vi "dIMU Complimentary Filter.vi"(7 "Port":T2 items=["Port 1", "Port 2", "Port 3", "Port 4"], 9 "Tau":dbl=3.0, 11 "NXT":T1) -> (0 "Yaw (deg)":dbl, 1 "Roll (deg)":dbl, 2 "Pitch (deg)":dbl, 3 "NXT":T1={"Hardware"="NXT", "Flattened String"=""})   [LabVIEW 2010]
uses:
  <vilib>/NXT/Block Support/NXT_InputPort.ctl
  <vilib>/NXT/Subs/LVHSConnector.ctl
  subVIs/dIMU_Accel_gs.vi
  subVIs/dIMU_Gyro_rads.vi
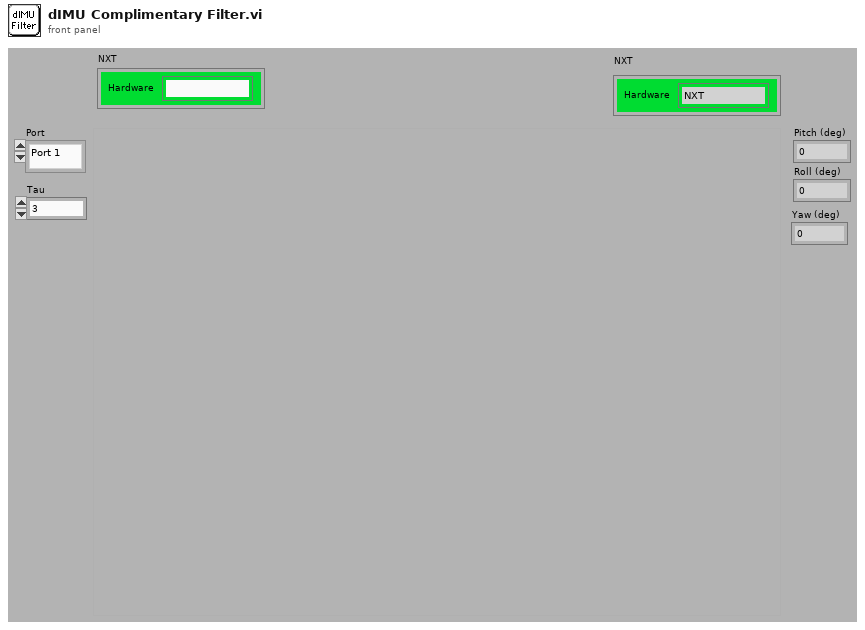
[diagram p1: front panel]
types:
  T1 = typedef "LVHSConnector.ctl" = cluster{"Hardware":string, "Flattened String":string}
  T2 = typedef "NXT_InputPort.ctl" = u8
  T3 = cluster{"Z Accel Offset":dbl, "Y Accel Offset":dbl, "X Accel Offset":dbl, "Z Gyro Offset":dbl, "Y Gyro Offset":dbl, "X Gyro Offset":dbl}
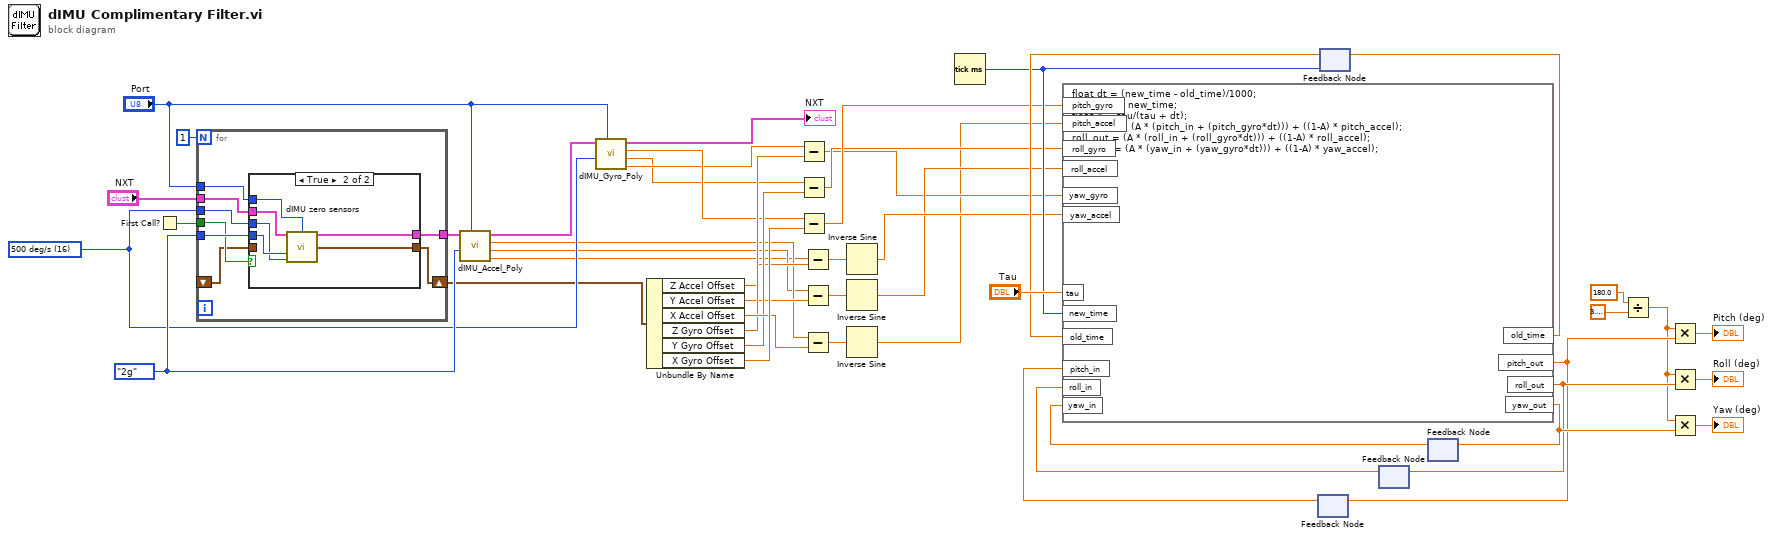
[diagram p0: block diagram]
diagram:
  w18 = u8 16 items=["250 deg/s"=0, "500 deg/s"=16, "2000 deg/s"=32] ("Gyro Scale")
  w24 = enum8{"2g", "4g", "8g"}."2g" ("Maximum Range")
  # "current axes are pitch (x) forward, roll (y) left, and yaw (z) up,\nshould these be rotated to standard aviation axes?"
  # "y = f(x) = A * y + (1-A) * x\nA = tau/(tau + dt)"
  n1 = First Call?() -> (First Call?: T/F=w17:bool)
  n2 = for {
    N: 1 -> [_]
    tunnel: "NXT" -> [w55]
    tunnel: [w54] -> w26
    tunnel: "Port" -> [w53]
    tunnel: w24 -> [w52]
    tunnel: w18 -> [w51]
    tunnel: w17 -> [w50]
    shift-right: [w49] -> w15
    shift-left: _ -> [w48]
    n3 = case shown="True" w50 {
      tunnel: w55 -> [w57 w63]
      tunnel: [w57 w62] -> w54
      tunnel: w53 -> [_ w61]
      tunnel: w52 -> [_ w60]
      tunnel: w51 -> [_ w59]
      tunnel: [w56 w58] -> w49
      tunnel: w48 -> [w56 _]
      frame False {
      }
      frame True {
        n4 = call "dIMU zero sensors.vi"("NXT 2"=w63, "Port"=w61, "Maximum Range"=w60, "Gyro Scale"=w59) -> ("NXT"=w62:T1, "Sensor Offsets"=w58:T3)  [unwired: 10 in]
      }
    }
  }
  n5 = call-poly "dIMU_Accel_Poly.vi"("Port"="Port", "Maximum Range"=w24, "NXT"=w26) -> ("Z Accel (g)"=w4:dbl, "Y Accel (g)"=w5:dbl, "X Accel (g)"=w6:dbl, "NXT"=w47:T1)  [unwired: 5 in]
  n6 = call-poly "dIMU_Gyro_Poly.vi"("Port"="Port", "Gyro Scale"=w18, "NXT"=w47) -> ("Z Gyro (rad/s"=w2:dbl, "Y Gyro (rad/s)"=w1:dbl, "X Gyro (rad/s)"=w3:dbl, "NXT"=→"NXT":T1)  [unwired: 5 in]
  n7 = Unbundle By Name(w15) -> ("Z Accel Offset"=w7:dbl, "Y Accel Offset"=w8:dbl, "X Accel Offset"=w12:dbl, "Z Gyro Offset"=w9:dbl, "Y Gyro Offset"=w10:dbl, "X Gyro Offset"=w14:dbl)
  n8 = Subtract(x=w2, y=w9) -> (x-y=w19:dbl)
  n9 = Subtract(x=w1, y=w10) -> (x-y=w20:dbl)
  n10 = Subtract(x=w3, y=w14) -> (x-y=w21:dbl)
  n11 = Subtract(x=w4, y=w7) -> (x-y=w22:dbl)
  n12 = Subtract(x=w5, y=w8) -> (x-y=w23:dbl)
  n13 = Subtract(x=w6, y=w12) -> (x-y=w11:dbl)
  n14 = Inverse Sine(1:w22) -> (0:w41:dbl)
  n15 = Inverse Sine(1:w23) -> (0:w40:dbl)
  n16 = Inverse Sine(1:w11) -> (0:w13:dbl)
  n17 = Tick Count (ms)() -> (millisecond timer value=w42:u32)
  n18 = feedback #1() -> (w29:dbl)  [unwired: 1 in]
  n19 = feedback #2(w42) -> (w43:dbl)
  n20 = feedback #3() -> (w31:dbl)  [unwired: 1 in]
  n21 = feedback #4() -> (w33:dbl)  [unwired: 1 in]
  n22 = formula code="float dt = (new_time - old_time)/1000;\nold_time = new_time;\nfloat A = tau/(tau + dt);\npitch_out = (A * (pitch_in + (pitch_gyro*dt))) + ((1-A) * pitch_accel);\nroll_out = (A * (roll_in + (roll_gyro*dt))) + ((1-A) * roll_accel);\nyaw_out = (A * (yaw_in + (yaw_gyro*dt))) + ((1-A) * yaw_accel);"("new_time"=w42, "tau"="Tau", "pitch_in"=w29, "pitch_gyro"=w21, "pitch_accel"=w13, "roll_gyro"=w20, "roll_accel"=w40, "roll_in"=w31, "yaw_in"=w33, "yaw_gyro"=w19, "yaw_accel"=w41, "old_time"=w43) -> ("pitch_out"=w30:dbl, "roll_out"=w32:dbl, "yaw_out"=w34:dbl, "old_time"=w44:dbl)
  n23 = feedback-in #1(w30) -> ()
  n24 = feedback-in #2(w44) -> ()
  n25 = feedback-in #3(w32) -> ()
  n26 = feedback-in #4(w34) -> ()
  n27 = Divide(x=180.0, y=3.141592653589793) -> (x/y=w28:dbl)
  n28 = Multiply(x=w28, y=w30) -> (x*y=→"Pitch (deg)":dbl)
  n29 = Multiply(x=w28, y=w32) -> (x*y=→"Roll (deg)":dbl)
  n30 = Multiply(x=w28, y=w34) -> (x*y=→"Yaw (deg)":dbl)
